vi "PLC.ChangeOver.vi"(7 "Idx":i32, 8 "error in":errorcluster, 10 "Slot":i32, 11 "Data_in":T1={"Status"={"Idx"=0, "ConnRef"=0, "State"=enum."Off", "LiveBitTimer"=timestamp(0 s since 1904-01-01)}, "Sets"={"Enable"=FALSE, "IP"="", "Rack"=0, "Slot"=0, "LifeBitTimer_s"=0.0, "DataBlockAddr_PCStatus"=0, "DataBlockAddr_PLCStatus"=1, "DataBlockAddr_PLCNewData"=[], "DataBlockSize_PLCNewData"=[], "DataBlockAddr_PLCChangeOver"=[], "DataBlockSize_PLCChangeOver"=[], "DataBlockAddr_PCChangeOver"=[], "DataBlockAddr_PLCCheckStatus"=[], "DataBlockSize_PLCCheckStatus"=[], "DataBlockAddr_PCCheckStatus"=[]}, "PCstatus"={"General"={"LifeBit"=FALSE, "DbRun"=FALSE}, "Stations"=[]}, "PLCstatus"={"General"={"LifeBit"=FALSE}, "Stations"=[]}}) -> (0 "error out":errorcluster, 3 "Data_out":T1={"Status"={"Idx"=0, "ConnRef"=0, "State"=enum."Off", "LiveBitTimer"=timestamp(0 s since 1904-01-01)}, "Sets"={"Enable"=FALSE, "IP"="", "Rack"=0, "Slot"=0, "LifeBitTimer_s"=0.0, "DataBlockAddr_PCStatus"=0, "DataBlockAddr_PLCStatus"=1, "DataBlockAddr_PLCNewData"=[], "DataBlockSize_PLCNewData"=[], "DataBlockAddr_PLCChangeOver"=[], "DataBlockSize_PLCChangeOver"=[], "DataBlockAddr_PCChangeOver"=[], "DataBlockAddr_PLCCheckStatus"=[], "DataBlockSize_PLCCheckStatus"=[], "DataBlockAddr_PCCheckStatus"=[]}, "PCstatus"={"General"={"LifeBit"=FALSE, "DbRun"=FALSE}, "Stations"=[]}, "PLCstatus"={"General"={"LifeBit"=FALSE}, "Stations"=[]}})   [LabVIEW 2016]
doc: "Get test results (measurement values) from PLC and save to database\n\nWabco 2017 All right reserved\nAuthor: maciej.szupienko@wabco-auto.com"
uses:
  PLC.Data.ctl
  PLC.Data.Status.ctl
  PLC.State.ctl
  PLC.Data.Sets.ctl
  LowLevel/PLC.DataBlock.PCstatus.ctl
  LowLevel/PLC.DataBlock.PCstatus.General.ctl
  LowLevel/PLC.DataBlock.PCstatus.Station.ctl
  LowLevel/PLC.DataBlock.PLCstatus.ctl
  LowLevel/PLC.DataBlock.PLCstatus.General.ctl
  LowLevel/PLC.DataBlock.PLCstatus.Station.ctl
  LowLevel/PLC.DataBlock.PLCchangeover.ctl
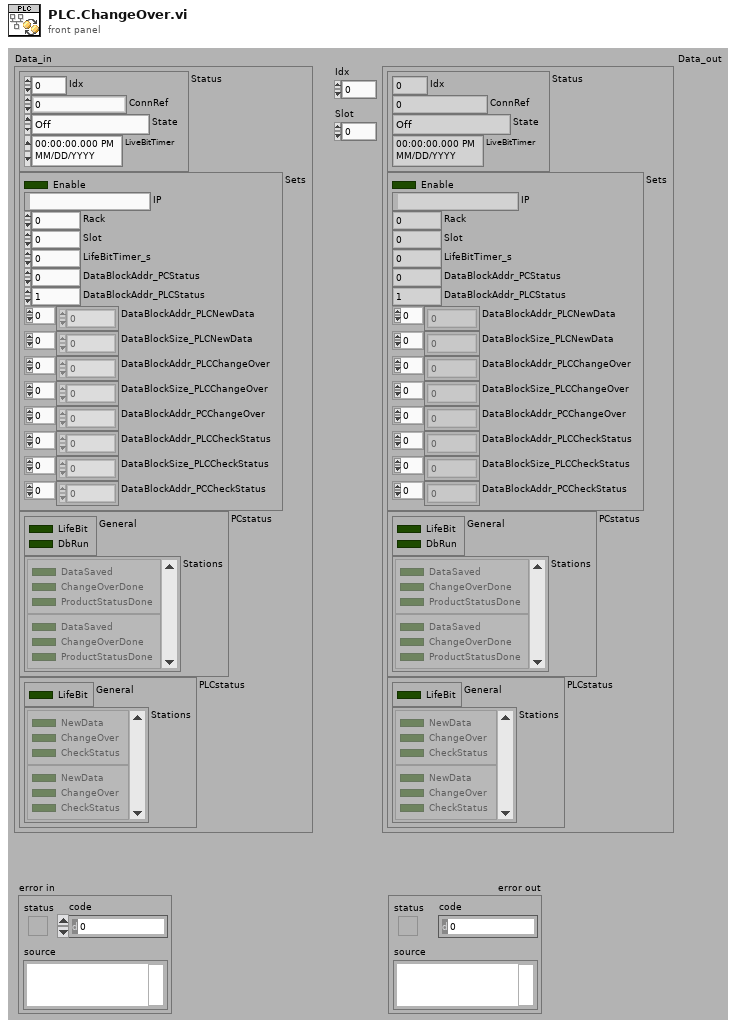
[diagram p1: front panel]
types:
  T1 = typedef "PLC.Data.ctl" = cluster{"Status":T2, "Sets":T4, "PCstatus":T5, "PLCstatus":T8}
  T2 = typedef "PLC.Data.Status.ctl" = cluster{"Idx":i32, "ConnRef":u64, "State":T3, "LiveBitTimer":timestamp}
  T3 = typedef "PLC.State.ctl" = enum32{"Off", "Error", "Idle", "Run"}
  T4 = typedef "PLC.Data.Sets.ctl" = cluster{"Enable":bool, "IP":string, "Rack":i32, "Slot":i32, "LifeBitTimer_s":dbl, "DataBlockAddr_PCStatus":i32, "DataBlockAddr_PLCStatus":i32, "DataBlockAddr_PLCNewData":i32[], "DataBlockSize_PLCNewData":i32[], "DataBlockAddr_PLCChangeOver":i32[], "DataBlockSize_PLCChangeOver":i32[], "DataBlockAddr_PCChangeOver":i32[], "DataBlockAddr_PLCCheckStatus":i32[], "DataBlockSize_PLCCheckStatus":i32[], "DataBlockAddr_PCCheckStatus":i32[]}
  T5 = typedef "PLC.DataBlock.PCstatus.ctl" = cluster{"General":T6, "Stations":T7[]}
  T6 = typedef "PLC.DataBlock.PCstatus.General.ctl" = cluster{"LifeBit":bool, "DbRun":bool}
  T7 = typedef "PLC.DataBlock.PCstatus.Station.ctl" = cluster{"DataSaved":bool, "ChangeOverDone":bool, "ProductStatusDone":bool}
  T8 = typedef "PLC.DataBlock.PLCstatus.ctl" = cluster{"General":T9, "Stations":T10[]}
  T9 = typedef "PLC.DataBlock.PLCstatus.General.ctl" = cluster{"LifeBit":bool}
  T10 = typedef "PLC.DataBlock.PLCstatus.Station.ctl" = cluster{"NewData":bool, "ChangeOver":bool, "CheckStatus":bool}
  T11 = typedef "PLC.DataBlock.PLCchangeover.ctl" = cluster{"Ref":string}
  T12 = typedef "PLC.DataBlock.PCchangeover.ctl" = cluster{"TP_Size":u8, "TV_Size":u8, "TP":sgl[], "TVL":sgl[], "TVH":sgl[]}
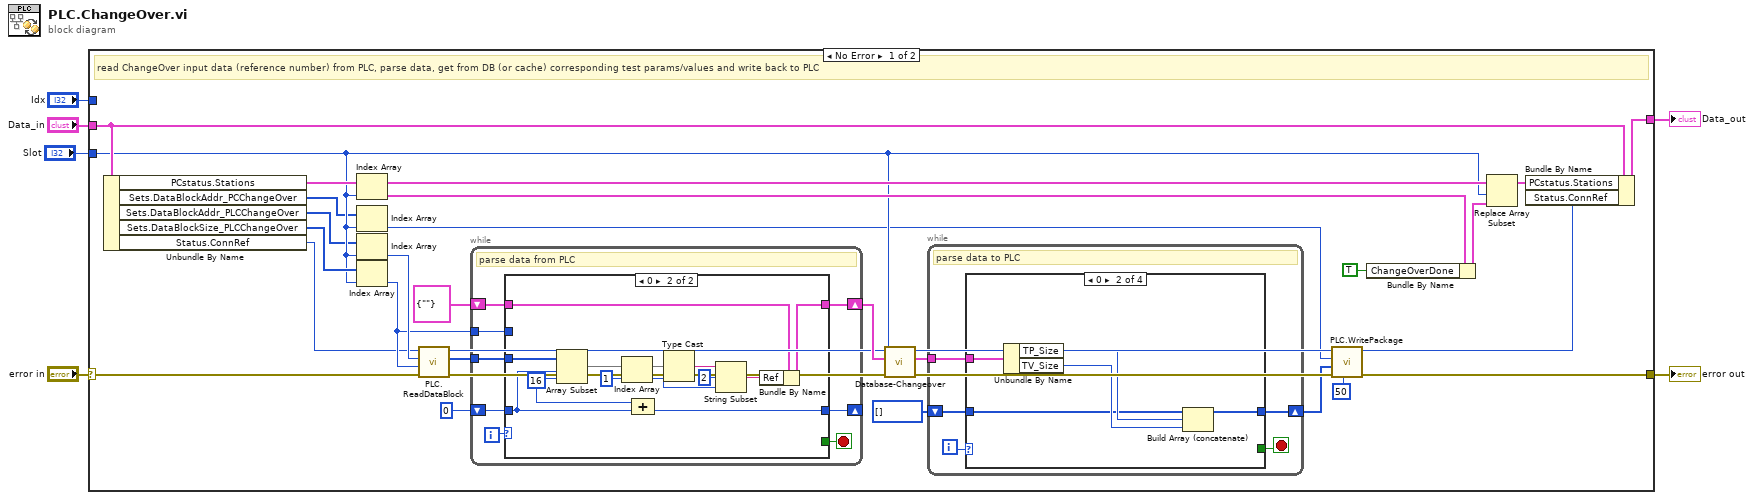
[diagram p0: block diagram]
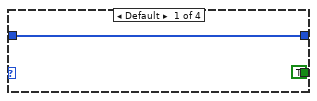
[diagram p2: hidden frame]
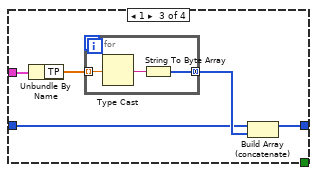
[diagram p3: hidden frame]
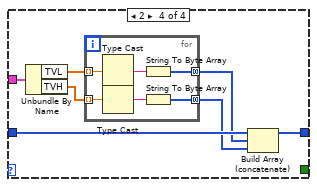
[diagram p4: hidden frame]
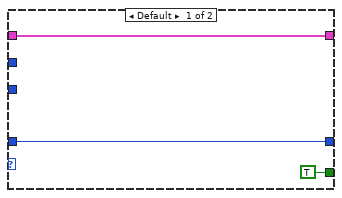
[diagram p5: hidden frame]
diagram:
  n1 = case shown="No Error" "error in" {
    selector: "error in" -> [w34 w93]
    tunnel: [w18 w93] -> w3
    tunnel: "Data_in" -> [w32 w92]
    tunnel: [w35 w92] -> w5
    tunnel: "Idx" -> [_ _]
    tunnel: "Slot" -> [w14 _]
    frame No Error {
      # "read ChangeOver input data (reference number) from PLC, parse data, get from DB (or cache) corresponding test params/values and write back to PLC"
      n2 = Unbundle By Name(w32) -> ("PCstatus.Stations"=w15:T7[], "Sets.DataBlockAddr_PCChangeOver"=w11:i32[], "Sets.DataBlockAddr_PLCChangeOver"=w12:i32[], "Sets.DataBlockSize_PLCChangeOver"=w22:i32[], "Status.ConnRef"=w10:u64)
      n3 = Index Array(array=w15, index=w14) -> (element=w30:T7)
      n4 = Index Array(array=w11, index=w14) -> (element=w9:i32)
      n5 = Index Array(array=w12, index=w14) -> (element=w33:i32)
      n6 = Index Array(array=w22, index=w14) -> (element=w24:i32)
      n7 = call "PLC.ReadDataBlock.vi"("error in (no error)"=w34, "Amount (1)"=w24, "Block"=w33, "Ref"=w10) -> ("error out"=w25:errorcluster, "data out"=w28:u8[], "ref out"=w19:u64)  [unwired: 5 in]
      n8 = while {
        tunnel: w28 -> [w71]
        shift-right: [w74] -> _
        shift-left: 0 -> [w75]
        shift-right: [w73] -> w23
        shift-left: T11 {"Ref"=""} ("element") -> [w72]
        tunnel: w24 -> [w70]
        i -> [w76]
        stop <- w69 stop-if-true
        # "parse data from PLC"
        n9 = case shown="0" w76 {
          tunnel: w75 -> [w78 w82]
          tunnel: [w78 w81] -> w74
          tunnel: [w79 w91] -> w73
          tunnel: w72 -> [w79 w90]
          tunnel: w71 -> [_ w85]
          tunnel: w70 -> [_ _]
          tunnel: [TRUE _] -> w69
          frame Default {
          }
          frame 0 {
            w83 = 16 ("length")
            n10 = Array Subset(array=w85, index=w82, length=w83) -> (w87:u8[])
            n11 = Index Array(array=w87, index=1) -> (element=w80:u8)
            n12 = Compound Arithmetic op=ADD(w83, w82) -> (w81:i32)
            n13 = Type Cast(x=w87) -> (*(type *) &x=w86:string)  [unwired: 1 in]
            n14 = String Subset(string=w86, offset (0)=2, length (rest)=w80) -> (substring=w84:string)
            n15 = Bundle By Name(cluster=w90, "Ref"=w84) -> (w91:T11)
          }
        }
      }
      n16 = call "Database-Changeover.vi"("error in"=w25, "PLCchangeover"=w23, "Idx"=w14) -> ("error out"=w21:errorcluster, "PCchangeover"=w20:T12)  [unwired: 7 in]
      n17 = while {
        tunnel: w20 -> [w39]
        shift-right: [w37] -> w8
        shift-left: u8[] [] ("data in") -> [w36]
        i -> [w40]
        stop <- w38 stop-if-true
        # "parse data to PLC"
        n18 = case shown="0" w40 {
          tunnel: w39 -> [_ w47 w52 w62]
          tunnel: [TRUE _ _ _] -> w38
          tunnel: [w41 w44 w48 w59] -> w37
          tunnel: w36 -> [w41 w43 w49 w60]
          frame Default {
          }
          frame 0 {
            n19 = Unbundle By Name(w47) -> ("TP_Size"=w46:u8, "TV_Size"=w45:u8)
            n20 = Build Array (concatenate)(w43, w46, w45) -> (w44:u8[])
          }
          frame 1 {
            n21 = Unbundle By Name(w52) -> ("TP"=w51:sgl[])
            n22 = for {
              tunnel: w51 -> [w55] mode=indexing
              tunnel: [w53] -> w50 mode=concatenating
              n23 = Type Cast(x=w55) -> (*(type *) &x=w54:string)  [unwired: 1 in]
              n24 = String To Byte Array(string=w54) -> (unsigned byte array=w53:u8[])
            }
            n25 = Build Array (concatenate)(w49, w50) -> (w48:u8[])
          }
          frame 2 {
            n26 = Unbundle By Name(w62) -> ("TVL"=w61:sgl[], "TVH"=w58:sgl[])
            n27 = for {
              tunnel: w61 -> [w68] mode=indexing
              tunnel: [w66] -> w56 mode=concatenating
              tunnel: w58 -> [w63] mode=indexing
              tunnel: [w65] -> w57 mode=concatenating
              n28 = Type Cast(x=w68) -> (*(type *) &x=w67:string)  [unwired: 1 in]
              n29 = Type Cast(x=w63) -> (*(type *) &x=w64:string)  [unwired: 1 in]
              n30 = String To Byte Array(string=w67) -> (unsigned byte array=w66:u8[])
              n31 = String To Byte Array(string=w64) -> (unsigned byte array=w65:u8[])
            }
            n32 = Build Array (concatenate)(w60, w56, w57) -> (w59:u8[])
          }
        }
      }
      n33 = call "PLC.WritePackage.vi"("max package size  (0: full)"=50 ("max package size  (0: all)"), "error in (no error)"=w21, "data"=w8, "addr"=w9, "Ref in"=w19) -> ("error out"=w18:errorcluster, "Ref out"=w16:u64)  [unwired: 5 in]
      n34 = Bundle By Name(cluster=w30, "ChangeOverDone"=TRUE) -> (w29:T7)
      n35 = Replace Array Subset(array=w15, new element=w29, index=w14) -> (w31:T7[])
      n36 = Bundle By Name(cluster=w32, "PCstatus.Stations"=w31, "Status.ConnRef"=w16) -> (w35:T1)
    }
    frame Error {
    }
  }
  "error out" <- w3
  "Data_out" <- w5
